vi "NO_NO_Auto_Routine_TestTrajectory.vi"(6 "End Orientation":dbl, 7 "Orientation":T1, 9 "Max Speed":dbl=7.0, 10 "Destination Waypoint":T2={"X"=60.0, "Y"=36.0, "ANGLE"=0.0, "WEIGHT"=2.0} {"WEIGHT" format="%13.3f"; "ANGLE" format="%13.3f"; "Y" format="%13.3f"; "X" format="%13.3f"}, 11 "Initial Waypoint":T2={"X"=0.0, "Y"=0.0, "ANGLE"=0.0, "WEIGHT"=2.0} {"WEIGHT" format="%13.3f"; "ANGLE" format="%13.3f"; "Y" format="%13.3f"; "X" format="%13.3f"}) -> ()   [LabVIEW 2023]
uses:
  <vilib>/Rock Robotics/WPI/ThirdParty/JAS_Junk/TrajLib/TypeDef/DISPLAY_WEIGHTED_WAYPOINT.ctl
  TrajectoryOrientation.ctl
  <vilib>/Rock Robotics/WPI/ThirdParty/JAS_Junk/TrajLib/Trajectory_Library.lvlib
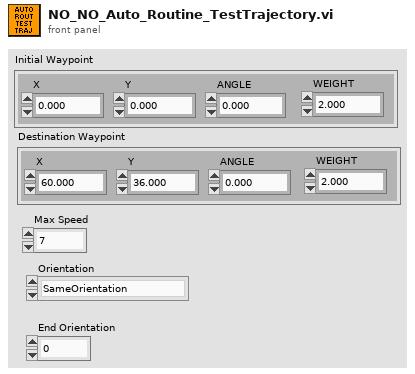
[diagram p1: front panel]
types:
  T1 = typedef "TrajectoryOrientation.ctl" = enum16{"SameOrientation", "RotateToEndOrientation"}
  T2 = typedef "Trajectory_Library.lvlib/DISPLAY_WEIGHTED_WAYPOINT.ctl" = cluster{"X":dbl, "Y":dbl, "ANGLE":dbl, "WEIGHT":dbl}
  T3 = typedef "Trajectory_Library.lvlib/TRAJECTORY.ctl" = cluster{"TotalTImeSecs":dbl, "States":T4[]}
  T4 = typedef "Trajectory_Library.lvlib/TRAJ_STATE.ctl" = cluster{"TimeSeconds":dbl, "Velocity":dbl, "Acceleration":dbl, "POSE":T5, "Curvature":dbl}
  T5 = typedef "Trajectory_Library.lvlib/POSE2D.ctl" = cluster{"TRANSLATION":T6, "ROTATION":T7}
  T6 = typedef "Trajectory_Library.lvlib/TRANSLATION2D.ctl" = cluster{"X":dbl, "Y":dbl}
  T7 = typedef "Trajectory_Library.lvlib/ROTATION2D.ctl" = cluster{"VALUE":dbl, "COS":dbl, "SIN":dbl}
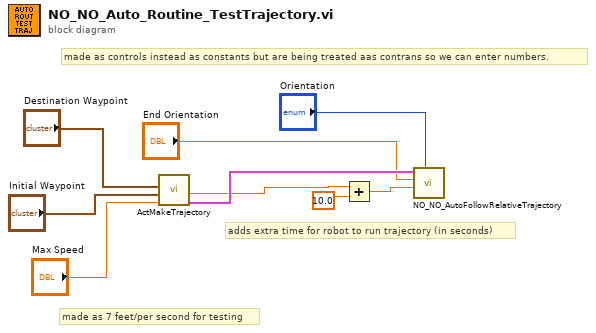
[diagram p0: block diagram]
diagram:
  # "made as controls instead as constants but are being treated aas contrans so we can enter numbers."
  # "made as 7 feet/per second for testing"
  # "adds extra time for robot to run trajectory (in seconds)"
  n1 = call "ActMakeTrajectory.vi"("Max Speed"="Max Speed", "Initial Waypoint"="Initial Waypoint", "Destination Waypoint"="Destination Waypoint") -> ("Absolute Trajectory"=w9:T3, "TotalTImeSecs"=w7:dbl)  [unwired: 5 in, 2 out]
  n2 = Add(x=w7, y=10.0) -> (x+y=w6:dbl)
  n3 = call "NO_NO_AutoFollowRelativeTrajectory.vi"("Orientation"="Orientation", "TimeOut (s)"=w6, "End Orientation"="End Orientation", "Trajectory"=w9) -> ()  [unwired: 7 in, 1 out]
